vi "Initialize Core.vi"(8 "error in (no error)":errorcluster, 10 "Parameters in":refnum<class "Abstract Init Parameters.lvclass">, 11 "Abstract Switch Consumer in":refnum<class "Abstract Switch Consumer.lvclass">) -> (0 "error out":errorcluster, 3 "Abstract Switch Consumer out":refnum<class "Abstract Switch Consumer.lvclass">)   [LabVIEW 2017, in "Messaging.lvlib" / "Abstract Switch Consumer.lvclass"]
uses:
  Abstract Switch Consumer.lvclass
  Parameters/Abstract Init Parameters/Abstract Init Parameters.lvclass
  Abstract Switch Init Parameters/Abstract Switch Init Parameters.lvclass
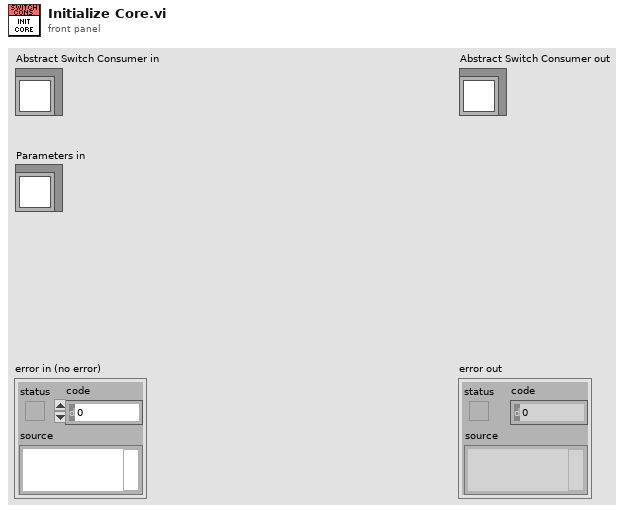
[diagram p1: front panel]
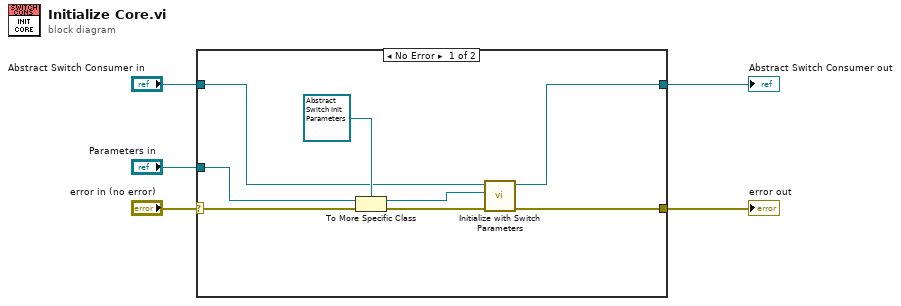
[diagram p0: block diagram]
diagram:
  n1 = case shown="No Error" "error in (no error)" {
    selector: "error in (no error)" -> [w6 w15]
    tunnel: [w10 w15] -> w5
    tunnel: [w9 w14] -> w4
    tunnel: "Abstract Switch Consumer in" -> [w8 w14]
    tunnel: "Parameters in" -> [w7 _]
    frame No Error {
      n2 = To More Specific Class(target class=refnum<class "Abstract Switch Init Parameters.lvclass"> refnum ("Message Queue Library.lvlib:Abstract Switch Init Parameters.lvclass"), reference=w7, error in=w6) -> (specific class reference=w12:refnum<class "Abstract Switch Init Parameters.lvclass">, error out=w11:errorcluster)
      n3 = call "Initialize with Switch Parameters.vi"("error in (no error)"=w11, "Switch Parameters in"=w12, "Abstract Switch Consumer in"=w8) -> ("error out"=w10:errorcluster, "Abstract Switch Consumer out"=w9:refnum<class "Abstract Switch Consumer.lvclass">)  [unwired: 7 in]
    }
    frame Error {
    }
  }
  "error out" <- w5
  "Abstract Switch Consumer out" <- w4
